vi "Boxcar filter2016.vi"(1 "Initialize":bool, 2 "Filter Size":i32, 3 "Filter Input":dbl format="%.2f") -> (0 "Filter Output":dbl format="%.2f")   [LabVIEW 2016]
uses:
  <vilib>/Analysis/baseanly.llb/Mean (DBL).vi
  <vilib>/Analysis/NI_AALBase.lvlib
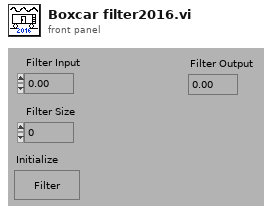
[diagram p1: front panel]
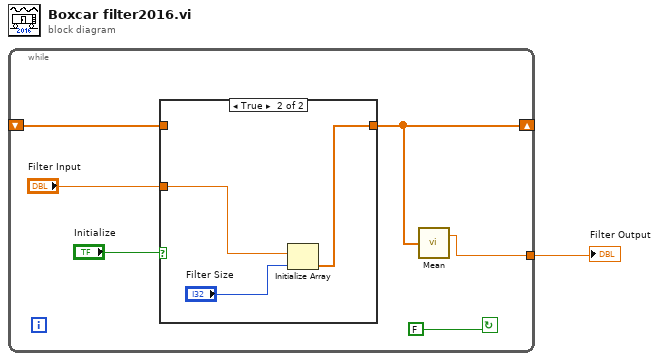
[diagram p0: block diagram]
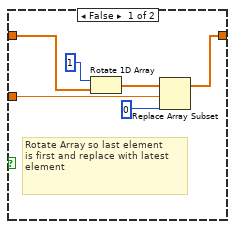
[diagram p2: hidden frame]
diagram:
  n1 = while {
    tunnel: [w2] -> w1
    shift-left: _ -> [w3]
    shift-right: [w4] -> _
    stop <- FALSE continue-if-true
    n2 = case shown="True" "Initialize" {
      tunnel: "Filter Input" -> [w9 w16]
      tunnel: [w11 w15] -> w4
      tunnel: w3 -> [w13 _]
      frame False {
        # "Rotate Array so last element \nis first and replace with latest element"
        n3 = Rotate 1D Array(1:w13, 2:1) -> (0:w10:dbl[])
        n4 = Replace Array Subset(array=w10, new element=w9, index=0) -> (w11:dbl[])
      }
      frame True {
        n5 = Initialize Array(w16, "Filter Size") -> (w15:dbl[])
      }
    }
    n6 = call-poly <vilib>:"Mean.vi"("X"=w4) -> ("mean"=w2:dbl)  [unwired: 1 out]
  }
  "Filter Output" <- w1
